vi "SpectrumCursor_set.vi"(0 "MapFunction":T1 items=["Total"=0, "Peak"=4, "Area"=2, "Value"=1, "Ratio"=3], 1 "Spectrum":refnum<vi>) -> ()   [LabVIEW 2010]
uses:
  _TypeDefs/MapFunctions.ctl
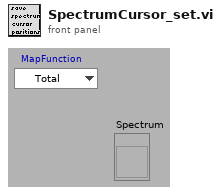
[diagram p1: front panel]
types:
  T1 = typedef "MapFunctions.ctl" = u16
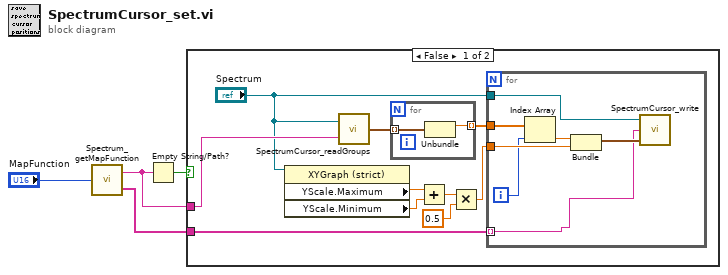
[diagram p0: block diagram]
diagram:
  n1 = call "Spectrum_getMapFunction.vi"("MapFunction"="MapFunction") -> ("CursorNames"=w3:string[], "Function"=w2:string)
  n2 = Empty String/Path?(string/path=w2) -> (empty?=w1:bool)
  n3 = case shown="False" w1 {
    tunnel: w2 -> [w6 _]
    tunnel: w3 -> [w8 _]
    frame False {
      n4 = property class="XYGraph (strict)"(reference="Spectrum") -> ("YScale.Maximum"=w12:dbl, "YScale.Minimum"=w13:dbl)  [unwired: 1 in, 2 out]
      n5 = call "SpectrumCursor_readGroups.vi"("first 4 letters from\ncursors group name"=w6, "graph ref"="Spectrum") -> ("cursors\npositions"=w10:cluster{"X":dbl, "Y":dbl}[])
      n6 = for {
        tunnel: w10 -> [w23] mode=indexing
        tunnel: [w22] -> w9 mode=indexing
        n7 = Unbundle(w23) -> ("X"=w22:dbl)  [unwired: 1 out]
      }
      n8 = Add(x=w12, y=w13) -> (x+y=w11:dbl)
      n9 = Multiply(x=w11, y=0.5) -> (x*y=w7:dbl)
      n10 = for {
        tunnel: w8 -> [w15] mode=indexing
        tunnel: w9 -> [w19]
        tunnel: w7 -> [w21]
        tunnel: "Spectrum" -> [w20]
        i -> [w18]
        n11 = Index Array(array=w19, index=w18) -> (element=w17:dbl)
        n12 = Bundle("X"=w17, w21) -> (w16:cluster{"X":dbl, dbl})  [unwired: 1 in]
        n13 = call "SpectrumCursor_write.vi"("cursor position"=w16, "existing\ncursor name"=w15, "graph ref"=w20) -> ()  [unwired: 1 in]
      }
    }
    frame True {
    }
  }
